vi "Load DAC Configuration.vi"(8 "error in":errorcluster, 10 "Config File refnum in":T1, 11 "DAC Heater Ctrl in":refnum<class "DAC Heater Ctrl.lvclass"> caption="DAC Heater dU in") -> (0 "error out":errorcluster, 2 "Config File refnum out":T1, 3 "DAC Heater Ctrl out":refnum<class "DAC Heater Ctrl.lvclass">)   [LabVIEW 2019, in "DAC.lvlib" / "DAC Heater Ctrl.lvclass"]
uses:
  DAC Heater Ctrl.lvclass
  <vilib>/Utility/config.llb/Config Data RefNum.ctl
  DAC.lvclass
  <vilib>/Utility/config.llb/NI_LVConfig.lvlib
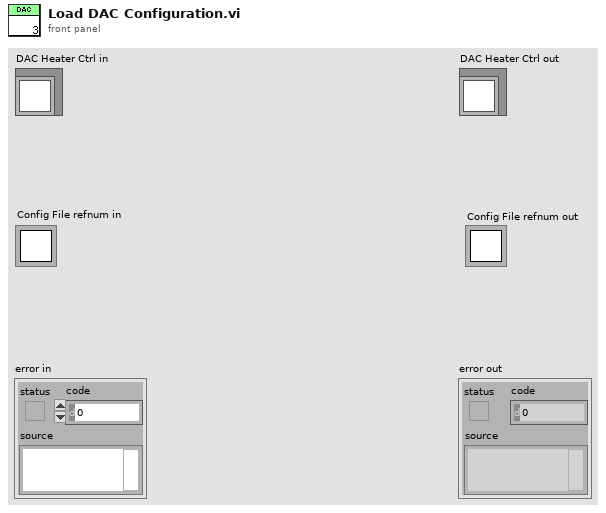
[diagram p1: front panel]
types:
  T1 = typedef "NI_LVConfig.lvlib/Config Data RefNum.ctl" = refnum<k1>
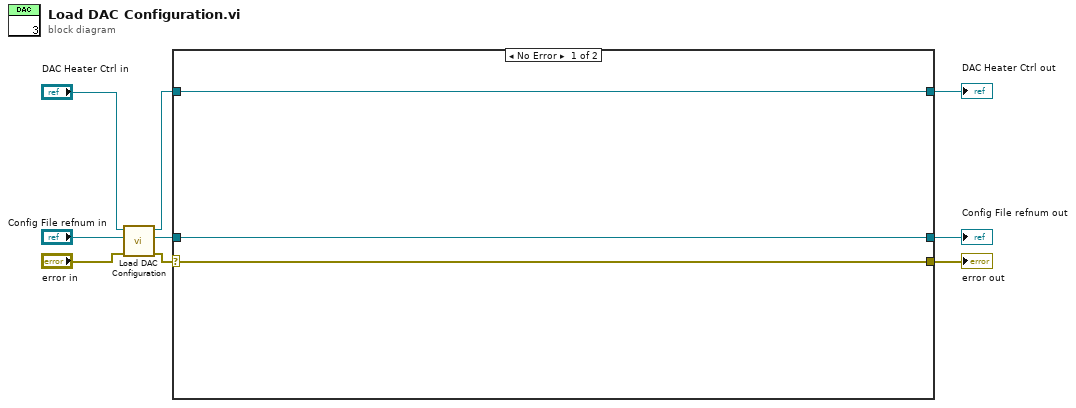
[diagram p0: block diagram]
diagram:
  n1 = call-parent "Load DAC Configuration.vi"("error in"="error in", "Config File refnum in"="Config File refnum in", "DAC in"="DAC Heater Ctrl in") -> ("error out"=w4:errorcluster, "Config File refnum out"=w5:T1, "DAC out"=w6:refnum<class "DAC Heater Ctrl.lvclass">)  [unwired: 6 in]
  n2 = case shown="No Error" w4 {
    selector: w4 -> [w11 w15]
    tunnel: [w11 w15] -> w1
    tunnel: [w10 w14] -> w3
    tunnel: w6 -> [w10 w14]
    tunnel: w5 -> [w12 w13]
    tunnel: [w12 w13] -> w2
    frame No Error {
    }
    frame Error {
    }
  }
  "error out" <- w1
  "DAC Heater Ctrl out" <- w3
  "Config File refnum out" <- w2
